vi "Periodic Tasks.vi"(8 "error in":errorcluster) -> ()   [LabVIEW 2013]
doc: "This VI runs in parallel to other tasks. It can contain as many user-defined periodic loops as you need. These can carry out PID or other sorts of timed response."
uses:
  RefnameEnum.ctl
  CollectorWrapAction.ctl
  DoubleSolenoidAction.ctl
  <vilib>/Rock Robotics/WPI/Compressor/WPI_CompressorGetSetRefNum.vi
  Robot Global Data.vi
  <vilib>/Rock Robotics/SystemInterfaces/Utilities/FPGA_UtilitiesLED Source.ctl
  <vilib>/Rock Robotics/SystemInterfaces/Utilities/FPGA_UtilitiesLED State.ctl
  SingleSolenoidAction.ctl
  TankDriveAction.ctl
  ShooterWrapperAction.ctl
  SonarAction.ctl
  AutoAlignMode.ctl
  CatchAction.ctl
  Example_Code/PressureSensor/PressureSensorAction.ctl
  ServoAction.ctl
panel:
  in  "CollectorMotorSpeed":dbl=1.0
  out "AutoDistanceWrapperIterations":i32=6512
  out "AutoDistanceWrapperTimer":u32=20
  in  "Slowdown":dbl=12.0 format="%#_13g"
  in  "Brake":dbl=6.0 format="%#_13g"
  in  "DesiredDistance":dbl=144.0 format="%#_13g"
  out "CatcherWrapperIterations":i32=2744
  out "CatcherWrapperTimer":u32=50
  out "CollectorWrapperTimer":u32=50
  out "CollectorWrapperIterations":i32=2743
  out "ShooterWrapperIterations":i32=2667
  out "ShooterWrapperTimer":u32=50
  out "CollectorIterations":i32=2737
  out "ClapperIterations":i32=2743
  out "RollerPneumaticIterations":i32=2743
  out "RollerMotorIterations":i32=2742
  out "FiringCylinderIterations":i32=2745
  out "KickerIterations":i32=2744
  out "SonicShifterIterations":i32=2744
  out "TankDriveIterations":i32=6485
  out "Collector Timer":u32=50
  out "Clapper Timer":u32=50
  out "Roller Pneumatic Timer":u32=50
  out "Firing Cylinder Timer":u32=50
  out "Sonic Shifter Timer":u32=50
  out "Kicker Timer":u32=50
  out "Roller Motor Timer":u32=51
  out "Tank Drive Timer":u32=21
  # "CATCH"
  # "SHOOTER WRAP"
  # "SONIC SHIFTER"
  # "TANK DRIVE"
  # "COLLECTOR WRAP"
  # "KICKER"
  # "ROLLER MOTOR"
  # "COLLECTOR ARM"
  # "FIRING CYLINDERS"
  # "AUTODISTANCE"
  # "ROLLER PNEUMATIC"
  # "CLAPPER"
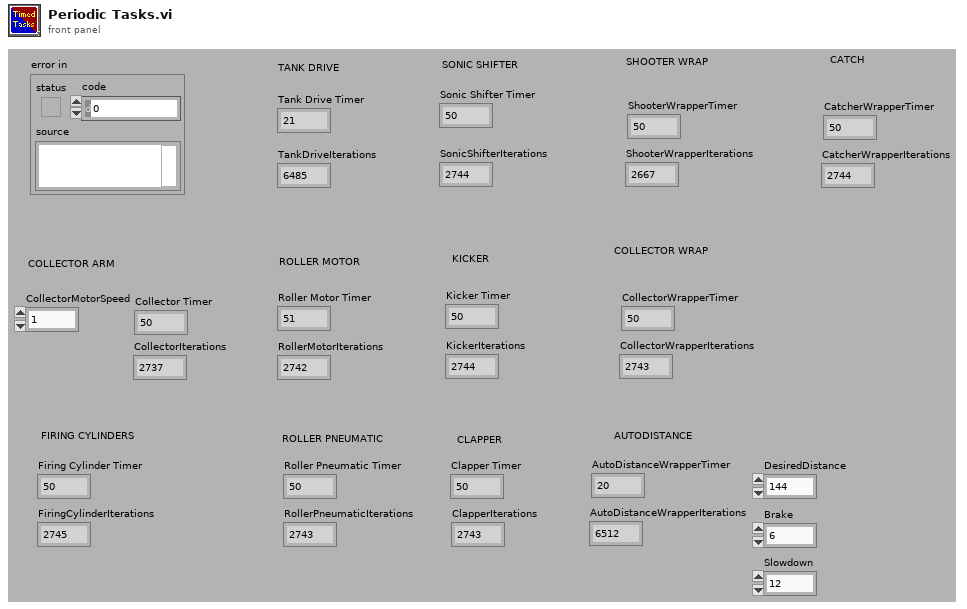
[diagram p1: front panel]
types:
  T1 = typedef "ShooterWrapperAction.ctl" = enum16{"Init", "CollectorDown", "CollectorUp"}
  T2 = typedef "CatchAction.ctl" = enum16{"PreCatch", "Catch", "Stop"}
  T3 = typedef "DoubleSolenoidAction.ctl" = enum16{"Init", "Middle", "In", "Out"}
  T4 = typedef "CollectorAction.ctl" = enum16{"Init", "Raise", "Lower", "Stop", "GetStatus"}
  T5 = typedef "CollectorWrapAction.ctl" = enum16{"PreCollect", "Collect", "Stop"}
  T6 = typedef "SingleSolenoidAction.ctl" = enum16{"Init", "SetState", "Disable"}
  T7 = typedef "TankDriveAction.ctl" = enum16{"Init", "LinearDrive", "SetValue", "Disable"}
  T8 = typedef "AutoAlignMode.ctl" = enum16{"Fullspeed", "Linear"}
  T9 = typedef "SonarAction.ctl" = enum16{"Init", "ReadValue", "Disable"}
  T10 = typedef "PressureSensorAction.ctl" = enum16{"Init", "ReadValue", "Disable"}
  T11 = typedef "ServoAction.ctl" = enum16{"Init", "SetAngle", "GetAngle", "Disable"}
  T12 = typedef "FPGA_UtilitiesLED State.ctl" = enum16{"Off", "On", "Toggle"}
  T13 = typedef "FPGA_UtilitiesLED Source.ctl" = enum16{"User LED", "FPGA LED"}
  T14 = typedef "RefnameEnum.ctl" = enum16{"TankDrive", "Controller1", "Controller2", "SonicShifter", "Compressor"}
  T15 = typedef "WPI_CompressorDevRef.ctl" = cluster{"DevStatus":errorcluster, "DigitalInputDevRef":T16, "RelayDevRef":T19}
  T16 = typedef "WPI_DigitalInputDevRef.ctl" = cluster{"DevStatus":errorcluster, "DIO Channel":T17, "Digital Module":T18}
  T17 = typedef "FPGA_DIOChannel.ctl" = enum8{"DIO 1", "DIO 2", "DIO 3", "DIO 4", "DIO 5", "DIO 6", "DIO 7", "DIO 8", "DIO 9", "DIO 10", "DIO 11", "DIO 12", "DIO 13", "DIO 14", "Invalid"}
  T18 = typedef "FPGA_TypedefDigitalModule.ctl" = enum16{"Digital Module 1", "Digital Module 2"}
  T19 = typedef "WPI_RelayDevRef.ctl" = cluster{"DevStatus":errorcluster, "Relay Channel":T20, "Digital Module":T18, "Relay Direction":T21}
  T20 = typedef "FPGA_DIORelayChannel.ctl" = enum8{"Relay 1", "Relay 2", "Relay 3", "Relay 4", "Relay 5", "Relay 6", "Relay 7", "Relay 8", "Invalid"}
  T21 = typedef "WPI_RelayDirection.ctl" = enum16{"Both directions", "Forward only", "Reverse only"}
  T22 = typedef "RollerAction.ctl" = enum16{"Init", "Off", "Forward", "Reverse"}
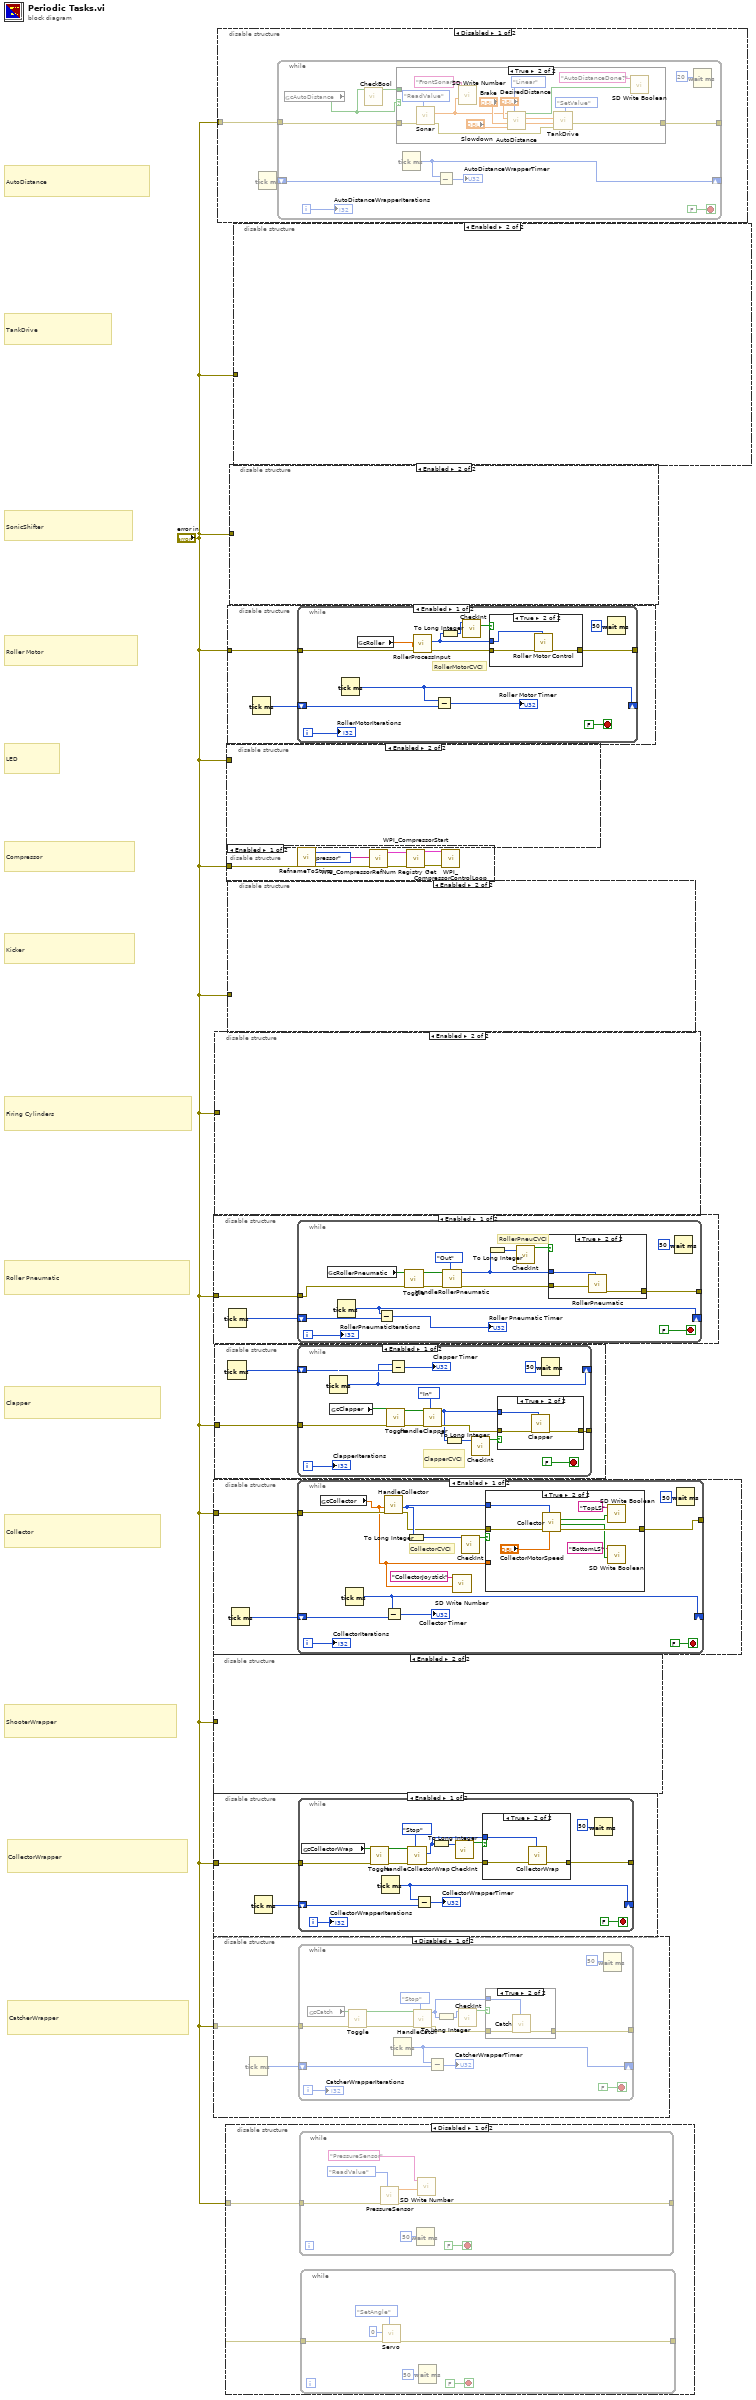
[diagram p0: block diagram]
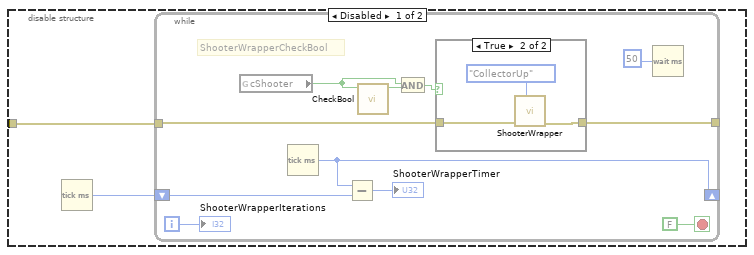
[diagram p7: hidden frame]
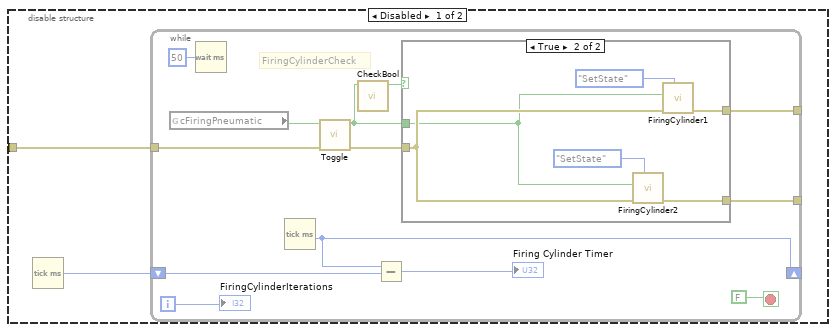
[diagram p15: hidden frame]
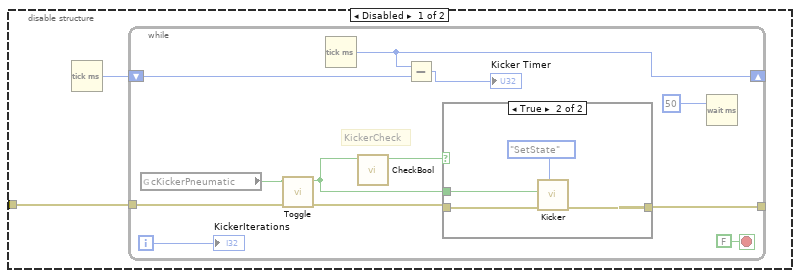
[diagram p17: hidden frame]
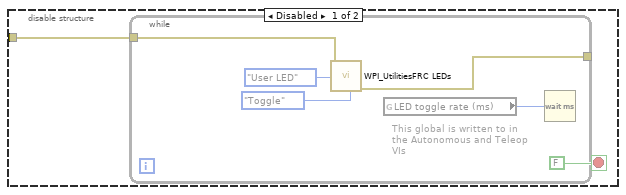
[diagram p20: hidden frame]
diagram:
  # "AutoDistance"
  # "CatcherWrapper"
  # "CollectorWrapper"
  # "ShooterWrapper"
  # "Collector"
  # "Clapper"
  # "Roller Pneumatic"
  # "Firing Cylinders"
  # "Kicker"
  # "Compressor"
  # "Roller Motor"
  # "SonicShifter"
  # "LED"
  # "TankDrive"
  n1 = disable-structure shown="Enabled" {
    disable-tunnel: "error in" -> [w3 _]
    frame Disabled {
      n2 = Tick Count (ms)() -> (millisecond timer value=w2:u32)
      n3 = while {
        tunnel: w3 -> [w10]
        shift-right: [w11] -> _
        shift-left: w2 -> [w12]
        tunnel: [w9] -> _
        i -> [w7]
        stop <- FALSE stop-if-true
        # "ShooterWrapperCheckBool"
        n4 = global read "Robot Global Data.vi" "cShooter"() -> (w4:bool)
        n5 = Tick Count (ms)() -> (millisecond timer value=w11:u32)
        n6 = Subtract(x=w11, y=w12) -> (x-y=→"ShooterWrapperTimer":u32)
        n7 = call "CheckBool.vi"("Input Boolean"=w4) -> ("Boolean Changed?"=w6:bool)  [unwired: 10 in]
        n8 = And(x=w4, y=w6) -> (x .and. y?=w5:bool)
        n9 = case shown="True" w5 {
          tunnel: w10 -> [w15 w18]
          tunnel: [w15 w17] -> w9
          frame False {
          }
          frame True {
            n10 = call "ShooterWrapper.vi"("Action"=ShooterWrapperAction."CollectorUp", "error in"=w18) -> ("error out"=w17:errorcluster)  [unwired: 8 in]
          }
        }
        n11 = Wait (ms)(milliseconds to wait=u32 50) -> ()  [unwired: 1 out]
        "ShooterWrapperIterations" <- w7
      }
    }
    frame Enabled {
    }
  }
  n12 = disable-structure shown="Disabled" {
    disable-tunnel: "error in" -> [w20 _]
    frame Disabled {
      n13 = Tick Count (ms)() -> (millisecond timer value=w19:u32)
      n14 = while {
        tunnel: w20 -> [w36]
        tunnel: [w33] -> _
        shift-right: [w28] -> _
        shift-left: w19 -> [w29]
        i -> [w30]
        stop <- FALSE stop-if-true
        n15 = global read "Robot Global Data.vi" "cCatch"() -> (w35:bool)
        n16 = call "Toggle.vi"("error in"=w36, "RawInput"=w35) -> ("error out"=w26:errorcluster, "ToggleState"=w22:bool)  [unwired: 8 in]
        n17 = Tick Count (ms)() -> (millisecond timer value=w28:u32)
        n18 = call "HandleCatch.vi"("InitState"=CatchAction."Stop", "error in (no error)"=w26, "Toggle?"=w22) -> ("error out"=w25:errorcluster, "State"=w23:T2)  [unwired: 7 in]
        n19 = Subtract(x=w28, y=w29) -> (x-y=→"CatcherWrapperTimer":u32)
        n20 = To Long Integer(number=w23) -> (32bit integer=w24:i32)
        n21 = call "CheckInt.vi"("Integer"=w24) -> ("Changed?"=w34:bool)  [unwired: 10 in]
        n22 = case shown="True" w34 {
          tunnel: w25 -> [w37 w40]
          tunnel: [w37 w39] -> w33
          tunnel: w23 -> [_ w38]
          frame False {
          }
          frame True {
            n23 = call "Catch.vi"("Action"=w38, "error in (no error)"=w40) -> ("error out"=w39:errorcluster)  [unwired: 9 in]
          }
        }
        n24 = Wait (ms)(milliseconds to wait=u32 50) -> ()  [unwired: 1 out]
        "CatcherWrapperIterations" <- w30
      }
    }
    frame Enabled {
    }
  }
  n25 = disable-structure shown="Enabled" {
    disable-tunnel: "error in" -> [w42 _]
    frame Enabled {
      n26 = Tick Count (ms)() -> (millisecond timer value=w41:u32)
      n27 = while {
        tunnel: w42 -> [w46]
        shift-right: [w55] -> _
        shift-left: w41 -> [w54]
        tunnel: [w48] -> _
        i -> [w47]
        stop <- FALSE stop-if-true
        # "RollerPneuCVCI"
        n28 = global read "Robot Global Data.vi" "cRollerPneumatic"() -> (w44:bool)
        n29 = Tick Count (ms)() -> (millisecond timer value=w55:u32)
        n30 = Subtract(x=w55, y=w54) -> (x-y=→"Roller Pneumatic Timer":u32)
        n31 = call "Toggle.vi"("error in"=w46, "RawInput"=w44) -> ("error out"=w45:errorcluster, "ToggleState"=w43:bool)  [unwired: 8 in]
        n32 = call "HandleRollerPneumatic.vi"("InitState"=DoubleSolenoidAction."Out", "error in (no error)"=w45, "Toggle?"=w43) -> ("error out"=w49:errorcluster, "State"=w50:T3)  [unwired: 7 in]
        n33 = To Long Integer(number=w50) -> (32bit integer=w52:i32)
        n34 = call "CheckInt.vi"("Integer"=w52) -> ("Changed?"=w51:bool)  [unwired: 10 in]
        n35 = case shown="True" w51 {
          tunnel: w50 -> [_ w62]
          tunnel: w49 -> [w59 w61]
          tunnel: [w59 w60] -> w48
          frame False {
          }
          frame True {
            n36 = call "RollerPneumatic.vi"("State"=w62, "Error in"=w61) -> ("Error out"=w60:errorcluster)  [unwired: 9 in]
          }
        }
        n37 = Wait (ms)(milliseconds to wait=u32 50) -> ()  [unwired: 1 out]
        "RollerPneumaticIterations" <- w47
      }
    }
    frame Disabled {
    }
  }
  n38 = disable-structure shown="Enabled" {
    disable-tunnel: "error in" -> [w64 _]
    frame Enabled {
      n39 = Tick Count (ms)() -> (millisecond timer value=w63:u32)
      n40 = while {
        tunnel: w64 -> [w77]
        shift-right: [w74] -> _
        shift-left: w63 -> [w75]
        tunnel: [w68] -> _
        i -> [w67]
        stop <- FALSE stop-if-true
        # "CollectorCVCI"
        n41 = global read "Robot Global Data.vi" "cCollector"() -> (w65:dbl)
        n42 = Tick Count (ms)() -> (millisecond timer value=w74:u32)
        n43 = call "HandleCollector.vi"("error in"=w77, "JoystickValue"=w65) -> ("error out"=w69:errorcluster, "CollectorEnum Input"=w70:T4)  [unwired: 8 in]
        n44 = Subtract(x=w74, y=w75) -> (x-y=→"Collector Timer":u32)
        n45 = To Long Integer(number=w70) -> (32bit integer=w72:i32)
        n46 = call <vilib>:"SD Write Number.vi"("Numeric"=w65, "Name"="CollectorJoystick") -> ()  [unwired: 8 in, 2 out]
        n47 = call "CheckInt.vi"("Integer"=w72) -> ("Changed?"=w71:bool)  [unwired: 10 in]
        n48 = case shown="True" w71 {
          tunnel: w70 -> [_ w87]
          tunnel: w69 -> [w79 w86]
          tunnel: [w79 w85] -> w68
          tunnel: w65 -> [_ _]
          frame False {
          }
          frame True {
            n49 = call "Collector.vi"("MotorSpeed"="CollectorMotorSpeed", "Action"=w87, "Error in"=w86) -> ("Error out"=w85:errorcluster, "Lower Triggered?"=w83:bool, "Upper Triggered?"=w84:bool)  [unwired: 6 in]
            n50 = call <vilib>:"SD Write Boolean.vi"("Boolean"=w84, "Name"="TopLS") -> ()  [unwired: 8 in, 2 out]
            n51 = call <vilib>:"SD Write Boolean.vi"("Boolean"=w83, "Name"="BottomLS") -> ()  [unwired: 8 in, 2 out]
          }
        }
        n52 = Wait (ms)(milliseconds to wait=u32 50) -> ()  [unwired: 1 out]
        "CollectorIterations" <- w67
      }
    }
    frame Disabled {
    }
  }
  n53 = disable-structure shown="Enabled" {
    disable-tunnel: "error in" -> [w89 _]
    frame Enabled {
      n54 = Tick Count (ms)() -> (millisecond timer value=w88:u32)
      n55 = while {
        tunnel: w89 -> [w98]
        shift-right: [w102] -> _
        shift-left: w88 -> [w103]
        tunnel: [w101] -> _
        i -> [w99]
        stop <- FALSE stop-if-true
        n56 = global read "Robot Global Data.vi" "cCollectorWrap"() -> (w97:bool)
        n57 = call "Toggle.vi"("error in"=w98, "RawInput"=w97) -> ("error out"=w96:errorcluster, "ToggleState"=w94:bool)  [unwired: 8 in]
        n58 = Tick Count (ms)() -> (millisecond timer value=w102:u32)
        n59 = call "HandleCollectorWrap.vi"("InitState"=CollectorWrapAction."Stop", "error in (no error)"=w96, "Toggle?"=w94) -> ("error out"=w93:errorcluster, "State"=w90:T5)  [unwired: 7 in]
        n60 = Subtract(x=w102, y=w103) -> (x-y=→"CollectorWrapperTimer":u32)
        n61 = To Long Integer(number=w90) -> (32bit integer=w91:i32)
        n62 = call "CheckInt.vi"("Integer"=w91) -> ("Changed?"=w92:bool)  [unwired: 10 in]
        n63 = case shown="True" w92 {
          tunnel: [w106 w109] -> w101
          tunnel: w93 -> [w106 w108]
          tunnel: w90 -> [_ w107]
          frame False {
          }
          frame True {
            n64 = call "CollectorWrap.vi"("Action"=w107, "error in"=w108) -> ("error out"=w109:errorcluster)  [unwired: 9 in]
          }
        }
        n65 = Wait (ms)(milliseconds to wait=u32 50) -> ()  [unwired: 1 out]
        "CollectorWrapperIterations" <- w99
      }
    }
    frame Disabled {
    }
  }
  n66 = disable-structure shown="Enabled" {
    disable-tunnel: "error in" -> [w111 _]
    frame Disabled {
      n67 = Tick Count (ms)() -> (millisecond timer value=w110:u32)
      n68 = while {
        tunnel: w111 -> [w116]
        shift-right: [w122] -> _
        shift-left: w110 -> [w121]
        tunnel: [w119] -> _
        tunnel: [w118] -> _
        i -> [w112]
        stop <- FALSE stop-if-true
        # "FiringCylinderCheck"
        n69 = global read "Robot Global Data.vi" "cFiringPneumatic"() -> (w117:bool)
        n70 = Wait (ms)(milliseconds to wait=u32 50) -> ()  [unwired: 1 out]
        n71 = Tick Count (ms)() -> (millisecond timer value=w122:u32)
        n72 = call "Toggle.vi"("error in"=w116, "RawInput"=w117) -> ("error out"=w115:errorcluster, "ToggleState"=w113:bool)  [unwired: 8 in]
        n73 = call "CheckBool.vi"("Input Boolean"=w113) -> ("Boolean Changed?"=w114:bool)  [unwired: 10 in]
        n74 = Subtract(x=w122, y=w121) -> (x-y=→"Firing Cylinder Timer":u32)
        n75 = case shown="True" w114 {
          tunnel: w115 -> [w125 w127]
          tunnel: [w125 w129] -> w119
          tunnel: [w125 w128] -> w118
          tunnel: w113 -> [_ w126]
          frame False {
          }
          frame True {
            n76 = call "FiringCylinder2.vi"("Action"=SingleSolenoidAction."SetState", "error in (no error)"=w127, "Actuate?"=w126) -> ("error out"=w128:errorcluster)  [unwired: 8 in]
            n77 = call "FiringCylinder1.vi"("Action"=SingleSolenoidAction."SetState", "error in (no error)"=w127, "Actuate?"=w126) -> ("error out"=w129:errorcluster)  [unwired: 8 in]
          }
        }
        "FiringCylinderIterations" <- w112
      }
    }
    frame Enabled {
    }
  }
  n78 = disable-structure shown="Enabled" {
    disable-tunnel: "error in" -> [w133 _]
    frame Enabled {
      n79 = Tick Count (ms)() -> (millisecond timer value=w132:u32)
      n80 = while {
        tunnel: w133 -> [w138]
        shift-right: [w134] -> _
        shift-left: w132 -> [w135]
        tunnel: [w144] -> _
        i -> [w140]
        stop <- FALSE stop-if-true
        # "ClapperCVCI"
        n81 = Tick Count (ms)() -> (millisecond timer value=w134:u32)
        n82 = global read "Robot Global Data.vi" "cClapper"() -> (w139:bool)
        n83 = call "Toggle.vi"("error in"=w138, "RawInput"=w139) -> ("error out"=w137:errorcluster, "ToggleState"=w136:bool)  [unwired: 8 in]
        n84 = Subtract(x=w134, y=w135) -> (x-y=→"Clapper Timer":u32)
        n85 = call "HandleClapper.vi"("InitState"=DoubleSolenoidAction."In", "error in (no error)"=w137, "Toggle?"=w136) -> ("error out"=w145:errorcluster, "State"=w142:T3)  [unwired: 7 in]
        n86 = To Long Integer(number=w142) -> (32bit integer=w143:i32)
        n87 = call "CheckInt.vi"("Integer"=w143) -> ("Changed?"=w141:bool)  [unwired: 10 in]
        n88 = case shown="True" w141 {
          tunnel: w142 -> [_ w153]
          tunnel: w145 -> [w150 w152]
          tunnel: [w150 w151] -> w144
          frame False {
          }
          frame True {
            n89 = call "Clapper.vi"("State"=w153, "Error in"=w152) -> ("Error out"=w151:errorcluster)  [unwired: 9 in]
          }
        }
        n90 = Wait (ms)(milliseconds to wait=u32 50) -> ()  [unwired: 1 out]
        "ClapperIterations" <- w140
      }
    }
    frame Disabled {
    }
  }
  n91 = disable-structure shown="Disabled" {
    disable-tunnel: "error in" -> [w155 _]
    frame Disabled {
      n92 = Tick Count (ms)() -> (millisecond timer value=w154:u32)
      n93 = while {
        tunnel: w155 -> [w165]
        tunnel: [w164] -> _
        shift-right: [w159] -> _
        shift-left: w154 -> [w160]
        i -> [w161]
        stop <- FALSE stop-if-true
        n94 = global read "Robot Global Data.vi" "cAutoDistance"() -> (w157:bool)
        n95 = call "CheckBool.vi"("Input Boolean"=w157) -> ("Boolean Changed?"=w156:bool)  [unwired: 10 in]
        n96 = case shown="True" w157 {
          tunnel: w165 -> [w168 w184]
          tunnel: [w167 w181] -> w164
          tunnel: w156 -> [w166 _]
          frame False {
            n97 = case shown="True" w166 {
              tunnel: w168 -> [w169 w173]
              tunnel: [w169 w172] -> w167
              frame False {
              }
              frame True {
                w171 = 0.0 ("LeftDesired")
                n98 = call "TankDrive.vi"("DriveAction"=TankDriveAction."SetValue", "error in (no error)"=w173, "RightDesired"=w171, "LeftDesired"=w171) -> ("error out"=w172:errorcluster)  [unwired: 6 in, 1 out]
              }
            }
          }
          frame True {
            n99 = call "Sonar.vi"("Action"=SonarAction."ReadValue", "error in (no error)"=w184) -> ("error out"=w178:errorcluster, "distance"=w180:dbl)  [unwired: 8 in]
            n100 = call <vilib>:"SD Write Number.vi"("Numeric"=w180, "Name"="FrontSonar") -> ()  [unwired: 8 in, 2 out]
            n101 = call "AutoDistance.vi"("Mode"=AutoAlignMode."Linear", "Slowdown"="Slowdown", "Brake"="Brake", "DesiredDistance"="DesiredDistance", "CurrentDistance"=w180) -> ("TankDriveRight"=w174:dbl, "TankDriveLeft"=w175:dbl, "Finished"=w177:bool)  [unwired: 4 in]
            n102 = call "TankDrive.vi"("DriveAction"=TankDriveAction."SetValue", "error in (no error)"=w178, "RightDesired"=w174, "LeftDesired"=w175) -> ("error out"=w181:errorcluster)  [unwired: 6 in, 1 out]
            n103 = call <vilib>:"SD Write Boolean.vi"("Boolean"=w177, "Name"="AutoDistanceDone?") -> ()  [unwired: 8 in, 2 out]
          }
        }
        n104 = Tick Count (ms)() -> (millisecond timer value=w159:u32)
        n105 = Subtract(x=w159, y=w160) -> (x-y=→"AutoDistanceWrapperTimer":u32)
        n106 = Wait (ms)(milliseconds to wait=u32 20) -> ()  [unwired: 1 out]
        "AutoDistanceWrapperIterations" <- w161
      }
    }
    frame Enabled {
    }
  }
  n107 = disable-structure shown="Disabled" {
    disable-tunnel: "error in" -> [w189 _]
    frame Disabled {
      n108 = while {
        tunnel: w189 -> [w195]
        tunnel: [w194] -> _
        stop <- FALSE stop-if-true
        n109 = call "PressureSensor.vi"("Action"=PressureSensorAction."ReadValue", "error in (no error)"=w195) -> ("error out"=w194:errorcluster, "Pressure"=w190:dbl)  [unwired: 8 in]
        n110 = Wait (ms)(milliseconds to wait=u32 50) -> ()  [unwired: 1 out]
        n111 = call <vilib>:"SD Write Number.vi"("Numeric"=w190, "Name"="PressureSensor") -> ()  [unwired: 8 in, 2 out]
      }
      n112 = while {
        tunnel: [w201] -> _
        tunnel: w189 -> [w199]
        stop <- FALSE stop-if-true
        n113 = call "Servo.vi"("Action"=ServoAction."SetAngle", "error in (no error)"=w199, "Angle (deg)"=0) -> ("error out"=w201:errorcluster)  [unwired: 7 in, 1 out]
        n114 = Wait (ms)(milliseconds to wait=u32 50) -> ()  [unwired: 1 out]
      }
    }
    frame Enabled {
    }
  }
  n115 = disable-structure shown="Enabled" {
    disable-tunnel: "error in" -> [w203 _]
    frame Disabled {
      n116 = while {
        tunnel: w203 -> [w205]
        tunnel: [w204] -> _
        stop <- FALSE stop-if-true
        # "This global is written to in the Autonomous and Teleop VIs"
        n117 = call <vilib>:"WPI_UtilitiesFRC LEDs.vi"("error in (no error)"=w205, "State"=FPGA_UtilitiesLED_State."Toggle", "LED Type"=FPGA_UtilitiesLED_Source."User LED") -> ("error out"=w204:errorcluster)  [unwired: 8 out]
        n118 = global read "Robot Global Data.vi" "LED toggle rate (ms)"() -> (w206:u32)
        n119 = Wait (ms)(milliseconds to wait=w206) -> ()  [unwired: 1 out]
      }
    }
    frame Enabled {
    }
  }
  n120 = disable-structure shown="Enabled" {
    disable-tunnel: "error in" -> [w216 _]
    frame Enabled {
      n121 = call "RefnameToString.vi"("Enum"=RefnameEnum."Compressor") -> ("Refname"=w213:string)
      n122 = call <vilib>:"WPI_CompressorRefNum Registry Get.vi"("error in (no error)"=w216, "refnum name"=w213) -> ("error out"=w215:errorcluster, "CompressorDevRef"=w211:T15)  [unwired: 8 in]
      n123 = call <vilib>:"WPI_CompressorStart.vi"("error in (no error)"=w215, "CompressorDevRef"=w211) -> ("error out"=w214:errorcluster, "CompressorDevRef"=w210:T15)  [unwired: 8 in]
      n124 = call <vilib>:"WPI_CompressorControlLoop.vi"("error in (no error)"=w214, "CompressorDevRef"=w210) -> ()  [unwired: 10 in]
    }
    frame Disabled {
    }
  }
  n125 = disable-structure shown="Enabled" {
    disable-tunnel: "error in" -> [w218 _]
    frame Enabled {
      n126 = Tick Count (ms)() -> (millisecond timer value=w217:u32)
      n127 = while {
        tunnel: w218 -> [w229]
        shift-right: [w227] -> _
        shift-left: w217 -> [w225]
        tunnel: [w221] -> _
        i -> [w219]
        stop <- FALSE stop-if-true
        # "RollerMotorCVCI"
        n128 = Tick Count (ms)() -> (millisecond timer value=w227:u32)
        n129 = global read "Robot Global Data.vi" "cRoller"() -> (w228:dbl)
        n130 = call "RollerProcessInput.vi"("error in"=w229, "JoystickValue"=w228) -> ("error out"=w222:errorcluster, "StateOut"=w220:T22)  [unwired: 8 in]
        n131 = Subtract(x=w227, y=w225) -> (x-y=→"Roller Motor Timer":u32)
        n132 = To Long Integer(number=w220) -> (32bit integer=w224:i32)
        n133 = call "CheckInt.vi"("Integer"=w224) -> ("Changed?"=w223:bool)  [unwired: 10 in]
        n134 = case shown="True" w223 {
          tunnel: w220 -> [_ w235]
          tunnel: w222 -> [w232 w234]
          tunnel: [w232 w233] -> w221
          frame False {
          }
          frame True {
            n135 = call "Roller Motor Control.vi"("Action"=w235, "Error in"=w234) -> ("Error out"=w233:errorcluster)  [unwired: 9 in]
          }
        }
        n136 = Wait (ms)(milliseconds to wait=u32 50) -> ()  [unwired: 1 out]
        "RollerMotorIterations" <- w219
      }
    }
    frame Disabled {
    }
  }
  n137 = disable-structure shown="Enabled" {
    disable-tunnel: "error in" -> [w237 _]
    frame Disabled {
      n138 = Tick Count (ms)() -> (millisecond timer value=w236:u32)
      n139 = while {
        tunnel: w237 -> [w243]
        shift-right: [w245] -> _
        shift-left: w236 -> [w247]
        tunnel: [w244] -> _
        i -> [w238]
        stop <- FALSE stop-if-true
        # "KickerCheck"
        n140 = global read "Robot Global Data.vi" "cKickerPneumatic"() -> (w241:bool)
        n141 = call "Toggle.vi"("error in"=w243, "RawInput"=w241) -> ("error out"=w242:errorcluster, "ToggleState"=w239:bool)  [unwired: 8 in]
        n142 = Tick Count (ms)() -> (millisecond timer value=w245:u32)
        n143 = call "CheckBool.vi"("Input Boolean"=w239) -> ("Boolean Changed?"=w240:bool)  [unwired: 10 in]
        n144 = Subtract(x=w245, y=w247) -> (x-y=→"Kicker Timer":u32)
        n145 = case shown="True" w240 {
          tunnel: w242 -> [w250 w252]
          tunnel: [w250 w253] -> w244
          tunnel: w239 -> [_ w251]
          frame False {
          }
          frame True {
            n146 = call "Kicker.vi"("Action"=SingleSolenoidAction."SetState", "error in (no error)"=w252, "Actuate?"=w251) -> ("error out"=w253:errorcluster)  [unwired: 8 in]
          }
        }
        n147 = Wait (ms)(milliseconds to wait=u32 50) -> ()  [unwired: 1 out]
        "KickerIterations" <- w238
      }
    }
    frame Enabled {
    }
  }
  n148 = disable-structure shown="Enabled" {
    disable-tunnel: "error in" -> [w256 _]
    frame Disabled {
      n149 = Tick Count (ms)() -> (millisecond timer value=w255:u32)
      n150 = while {
        tunnel: w256 -> [w261]
        shift-right: [w265] -> _
        shift-left: w255 -> [w266]
        tunnel: [w263] -> _
        i -> [w258]
        stop <- FALSE stop-if-true
        n151 = global read "Robot Global Data.vi" "cSonicShifter"() -> (w262:bool)
        n152 = call "Toggle.vi"("error in"=w261, "RawInput"=w262) -> ("error out"=w260:errorcluster, "ToggleState"=w257:bool)  [unwired: 8 in]
        n153 = Tick Count (ms)() -> (millisecond timer value=w265:u32)
        n154 = Subtract(x=w265, y=w266) -> (x-y=→"Sonic Shifter Timer":u32)
        n155 = call "CheckBool.vi"("Input Boolean"=w257) -> ("Boolean Changed?"=w259:bool)  [unwired: 10 in]
        n156 = case shown="True" w259 {
          tunnel: [w269 w272] -> w263
          tunnel: w260 -> [w269 w271]
          tunnel: w257 -> [_ w270]
          frame False {
          }
          frame True {
            n157 = call "SonicShifter.vi"("Action"=SingleSolenoidAction."SetState" ("Mode"), "error in (no error)"=w271, "Actuate?"=w270) -> ("error out"=w272:errorcluster)  [unwired: 8 in]
          }
        }
        n158 = Wait (ms)(milliseconds to wait=u32 50) -> ()  [unwired: 1 out]
        "SonicShifterIterations" <- w258
      }
    }
    frame Enabled {
    }
  }
  n159 = disable-structure shown="Enabled" {
    disable-tunnel: "error in" -> [w275 _]
    frame Disabled {
      n160 = Tick Count (ms)() -> (millisecond timer value=w274:u32)
      n161 = while {
        tunnel: w275 -> [w280]
        shift-right: [w299] -> _
        shift-left: w274 -> [w298]
        tunnel: [w291] -> _
        i -> [w288]
        stop <- FALSE stop-if-true
        n162 = global read "Robot Global Data.vi" "cReverseDrive"() -> (w287:bool)
        n163 = global read "Robot Global Data.vi" "cStraightDrive"() -> (w284:bool)
        n164 = global read "Robot Global Data.vi" "cTankDriveRight"() -> (w296:dbl)
        n165 = global read "Robot Global Data.vi" "cTankDriveLeft"() -> (w295:dbl)
        n166 = global read "Robot Global Data.vi" "cHalfDrive"() -> (w283:bool)
        n167 = Tick Count (ms)() -> (millisecond timer value=w299:u32)
        n168 = Wait (ms)(milliseconds to wait=u32 20) -> ()  [unwired: 1 out]
        n169 = call "Toggle.vi"("RawInput"=w287) -> ("ToggleState"=w281:bool)  [unwired: 9 in, 1 out]
        n170 = Subtract(x=w299, y=w298) -> (x-y=→"Tank Drive Timer":u32)
        n171 = call "Sonar.vi"("Action"=SonarAction."ReadValue", "error in (no error)"=w280) -> ("error out"=w278:errorcluster, "distance"=w276:dbl)  [unwired: 8 in]
        n172 = call "HandleDrive.vi"("Deadzone"=0.15, "RightMotor"=w296, "LeftMotor"=w295) -> ("Enqueue?"=w294:bool, "RightMotor"=w292:dbl, "LeftMotor"=w293:dbl)  [unwired: 6 in]
        n173 = call <vilib>:"SD Write Boolean.vi"("Boolean"=w281, "Name"="ReverseDrive") -> ()  [unwired: 8 in, 2 out]
        n174 = call <vilib>:"SD Write Number.vi"("error in"=w278, "Numeric"=w276, "Name"="FrontSonar") -> ()  [unwired: 7 in, 2 out]
        n175 = call <vilib>:"SD Write Boolean.vi"("Boolean"=w284, "Name"="StraightDrive") -> ()  [unwired: 8 in, 2 out]
        n176 = call <vilib>:"SD Write Boolean.vi"("Boolean"=w283, "Name"="HalfDrive") -> ()  [unwired: 8 in, 2 out]
        n177 = case shown="True" w294 {
          tunnel: w293 -> [_ w310]
          tunnel: w292 -> [_ w309]
          tunnel: [w301 w308] -> w291
          tunnel: w280 -> [w301 w307]
          tunnel: w281 -> [_ w304]
          tunnel: w283 -> [_ w303]
          tunnel: w284 -> [_ w302]
          frame False {
          }
          frame True {
            w317 = 0.0  # Cutoff
            n178 = call "HalfDrive.vi"("RightDrive in"=w309, "LeftDrive in"=w310, "HalfDrive"=w303) -> ("RightDrive out"=w316:dbl, "LeftDrive out"=w315:dbl)  [unwired: 7 in]
            n179 = call "StraightDrive.vi"("RightDrive in"=w316, "LeftDrive in"=w315, "StraightDrive"=w302) -> ("RightDrive out"=w313:dbl, "LeftDrive out"=w314:dbl)  [unwired: 7 in]
            n180 = call "ReverseDrive.vi"("cReverseDrive"=w304, "Right"=w313, "Left"=w314) -> ("Right"=w311:dbl, "Left"=w312:dbl)  [unwired: 7 in]
            n181 = call <vilib>:"SD Read Number.vi"("Name"="MaxMotorChange") -> ("Numeric"=w305:dbl)  [unwired: 8 in, 2 out]
            n182 = call "TankDrive.vi"("MaxMotorChangeForward"=w305, "Cutoff"=w317, "DriveAction"=TankDriveAction."SetValue", "error in (no error)"=w307, "RightDesired"=w311, "LeftDesired"=w312) -> ("error out"=w308:errorcluster)  [unwired: 4 in, 1 out]
          }
        }
        "TankDriveIterations" <- w288
      }
    }
    frame Enabled {
    }
  }
